vi "ATS_Initialize.vi"(10 "PreSet_Device":bool, 11 "Device":i32) -> (0 "Code":i32, 2 "#System":i32, 3 "DeviceOut":i32)   [LabVIEW 2010]
doc: "_____AlazarTech, Scope_____\n\nInitialize board and control.\n\nInput:\n\n\"PreSet_Device\" :\n -True: the device will be initialize to a Preset state.\n -False: no setting will be made on the device. The board will be in an unknown state for LabVIEW.\n\nOutput:\n\n\"DeviceOut\": same as Device\n\"#System\": number of system found.\n\"Code\" : error if any. No Error = 512"
uses:
  ATS_ctl/ATS_Global_Ctrl.ctl
  ATS_ctl/ATS_Cards_GBL.vi
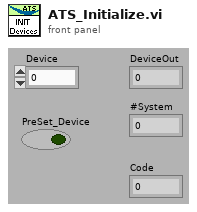
[diagram p1: front panel]
types:
  T1 = typedef "Device_Info.ctl" = cluster{"Handle":u32, "Board":string, "CPLD":string, "MemorySize":u32, "SampleSize":u8, "ID":i32, "High_Memory":bool, "Chan/Board":u8}
  T2 = typedef "ATS_Global_Ctrl.ctl" = enum16{"Init_Device", "Clear_ALL", "Set", "Get"}
  T3 = typedef "ATS_Global_4Ch.ctl" = cluster{"Record":T4, "Clock":T5, "Inputs":T9, "Trigger":T15}
  T4 = typedef "Record.ctl" = cluster{"Count":u32, "Presize":u32, "Length":u32}
  T5 = typedef "Clock.ctl" = cluster{"ClckSource":T6, "ClckRate":T7, "ClckEdge":T8, "Decimation":u32}
  T6 = typedef "ClockSource.ctl" = enum16{"Internal", "External", "Medium Ext.", "Slow Ext.", "Ext. AC", "Ext. DC", "Ext. (PLL)"}
  T7 = typedef "ClockRate.ctl" = u32
  T8 = typedef "ClockEdge.ctl" = u16
  T9 = typedef "ATS_InputArray.ctl" = T10[]
  T10 = typedef "InputCtrl.ctl" = cluster{"Coupling":T11, "Range":T12, "Impedance":T13, "Bandwidth":T14}
  T11 = typedef "Coupling.ctl" = enum16{"AC", "DC"}
  T12 = typedef "Range.ctl" = u32
  T13 = typedef "Impedance.ctl" = enum16{"1M ohms", "50 ohms"}
  T14 = typedef "Bandwidth.ctl" = enum16{"Full Bandwidth", "Reduce Bandwidth"}
  T15 = typedef "ATS_Trigger_4Ch.ctl" = cluster{"TrigOperation":T16, "Timeout (s)":dbl, "Trig. Delay":u32, "Engine X":T17, "Engine Y":T17, "ExtTrigControl":T19}
  T16 = typedef "TriggerOperation.ctl" = enum16{"Only X", "Only Y", "X or Y", "X and Y", "X xor Y", "X and not Y", "not X and Y"}
  T17 = typedef "ATS_TriggerEngine_4Ch.ctl" = cluster{"Source":T18, "Slope":enum32{"Positive", "Negative"}, "Level":u32}
  T18 = typedef "ATS_TriggerSource_4Ch.ctl" = enum32{"Chan_A", "Chan_B", "External", "Disable", "Chan_C", "Chan_D"}
  T19 = typedef "ExtTrigger.ctl" = cluster{"Coupling":T11, "Range":T20}
  T20 = typedef "ExtTrigRange.ctl" = enum16{"1 V", "5 V", "TTL"}
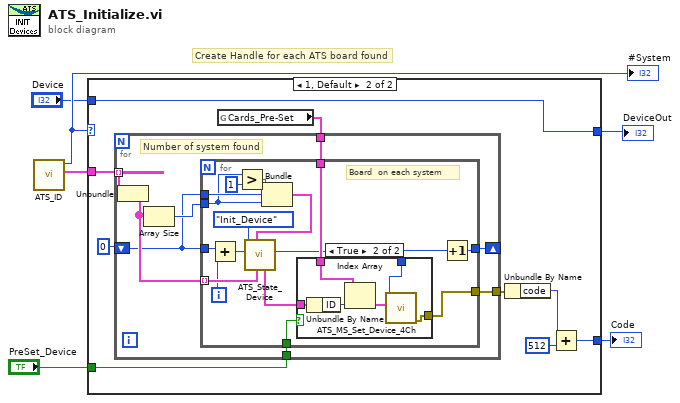
[diagram p0: block diagram]
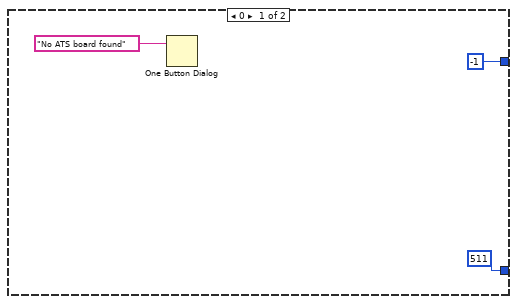
[diagram p2: hidden frame]
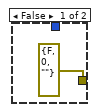
[diagram p3: hidden frame]
diagram:
  # "Create Handle for each ATS board found"
  n1 = call "ATS_ID.vi"() -> ("ATS_System"=w6:cluster{"System":u32, "Devices":T1[]}[], "#System"=w5:i32)  [unwired: 5 in, 1 out]
  "#System" <- w5
  n2 = case shown="1, Default" w5 {
    tunnel: "Device" -> [_ w13]
    tunnel: [-1 ("#Device") w13] -> w3
    tunnel: w6 -> [_ w15]
    tunnel: "PreSet_Device" -> [_ w12]
    tunnel: [511 ("Handle") w11] -> w1
    frame 0 {
      n3 = One Button Dialog(message="No ATS board found") -> ()  [unwired: 1 in, 1 out]
    }
    frame 1, Default {
      n4 = global read "ATS_Cards_GBL.vi" "Cards_Pre-Set"() -> (w10:T3[])
      n5 = for {
        tunnel: [w26] -> w18
        tunnel: w10 -> [w25]
        tunnel: w15 -> [w24] mode=indexing
        shift-right: [w20] -> _
        shift-left: 0 -> [w21]
        tunnel: w12 -> [w19]
        # "Number of system found"
        n6 = Unbundle(w24) -> ("Devices"=w23:T1[])  [unwired: 1 out]
        n7 = Array Size(array=w23) -> (size(s)=w22:i32)
        n8 = for {
          tunnel: [w41] -> w26
          tunnel: w23 -> [w38] mode=indexing
          tunnel: w25 -> [w40]
          tunnel: w22 -> [w34]
          tunnel: w21 -> [w37]
          tunnel: w21 -> [w30]
          tunnel: [w28] -> w20
          tunnel: w19 -> [w27]
          i -> [w31]
          # "Board  on each system"
          n9 = Add(x=w30, y=w31) -> (x+y=w32:i32)
          n10 = Greater?(x=w34, y=1) -> (0:w36:bool)
          n11 = Bundle(w36, w37, w34) -> (w35:cluster{bool, i32, i32})  [unwired: 1 in]
          n12 = call "ATS_State_Device.vi"("DevInfo_In"=w38, "Sys_In"=w35, "DeviceIn"=w32, "ATS_GBL_Ctrl"=ATS_Global_Ctrl."Init_Device") -> ("DeviceOut"=w29:i32, "DevInfo_Out"=w39:T1)  [unwired: 2 in, 4 out]
          n13 = case shown="True" w27 {
            tunnel: [errorcluster {"status"=FALSE, "code"=0, "source"=""} ("error out") w49] -> w41
            tunnel: w40 -> [_ w48]
            tunnel: w39 -> [_ w47]
            tunnel: w29 -> [_ w46]
            frame False {
            }
            frame True {
              n14 = Unbundle By Name(w47) -> ("ID"=w45:i32)
              n15 = Index Array(array=w48, index=w45) -> (element=w44:T3)
              n16 = call "ATS_MS_Set_Device_4Ch.vi"("Setup_In"=w44, "DeviceIn"=w46) -> ("error out"=w49:errorcluster)  [unwired: 4 in, 5 out]
            }
          }
          n17 = Increment(x=w29) -> (x+1=w28:i32)
        }
      }
      n18 = Unbundle By Name(w18) -> ("code"=w17:i32)
      n19 = Add(x=w17, y=512) -> (x+y=w11:i32)
    }
  }
  "DeviceOut" <- w3
  "Code" <- w1
